vi "Begin.vi"(11 "Image Size":T1=enum."160x120") -> (0 "error out":errorcluster)   [LabVIEW 2012]
doc: "Called before other user functions, this VI is expected to open initial I/O refnums, load in file data, and do all program initialization. Notice that the <B>error out</B> terminal is simply used for data flow. Wiring it to other structures or subVIs ensures that this VI runs first."
uses:
  <vilib>/Rock Robotics/WPI/Camera/WPI_CameraImageSize.ctl
  <vilib>/Rock Robotics/WPI/Camera/WPI_CameraWhite Balance Values.ctl
  <vilib>/Rock Robotics/WPI/Camera/WPI_CameraExposure Values.ctl
  <vilib>/Rock Robotics/WPI/Camera/WPI_CameraFrameRate.ctl
  <vilib>/Rock Robotics/WPI/DriverStation/WPI_DriverStationRobotMode2.ctl
  <vilib>/Rock Robotics/SystemInterfaces/DIO/FPGA_DIOPWMChannel.ctl
  <vilib>/Rock Robotics/WPI/Joystick/WPI_JoystickDeviceEnum.ctl
  <vilib>/Rock Robotics/SystemInterfaces/Typedef/FPGA_TypedefDigitalModule.ctl
  <vilib>/Rock Robotics/WPI/Relay/WPI_RelayDirection.ctl
  <vilib>/Rock Robotics/SystemInterfaces/DIO/FPGA_DIORelayChannel.ctl
  <vilib>/Rock Robotics/SystemInterfaces/AI/FPGA_AIChannel.ctl
  <vilib>/Rock Robotics/SystemInterfaces/AI/FPGA_AIGyroChannel.ctl
  <vilib>/Rock Robotics/SystemInterfaces/DIO/FPGA_DIOChannel.ctl
  Robot Global Data.vi
  <vilib>/Rock Robotics/WPI/MotorControl/WPI_MotorControlOpen Victor.vi
  <vilib>/Rock Robotics/WPI/MotorControl/WPI_MotorControlOpen Jaguar.vi
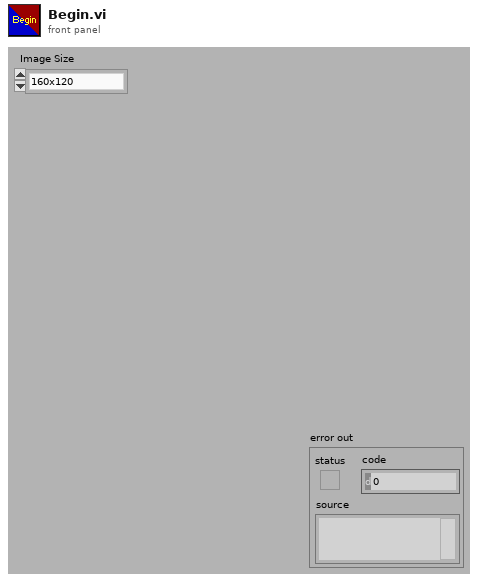
[diagram p1: front panel]
types:
  T1 = typedef "WPI_CameraImageSize.ctl" = enum16{"640x480", "320x240", "160x120"}
  T2 = typedef "FPGA_AIChannel.ctl" = enum8{"AI 1", "AI 2", "AI 3", "AI 4", "AI 5", "AI 6", "AI 7", "AI 8", "Invalid"}
  T3 = typedef "FPGA_DIOChannel.ctl" = enum8{"DIO 1", "DIO 2", "DIO 3", "DIO 4", "DIO 5", "DIO 6", "DIO 7", "DIO 8", "DIO 9", "DIO 10", "DIO 11", "DIO 12", "DIO 13", "DIO 14", "Invalid"}
  T4 = typedef "FPGA_TypedefDigitalModule.ctl" = enum16{"Digital Module 1", "Digital Module 2"}
  T5 = typedef "FPGA_DIOPWMChannel.ctl" = enum8{"PWM 1", "PWM 2", "PWM 3", "PWM 4", "PWM 5", "PWM 6", "PWM 7", "PWM 8", "PWM 9", "PWM 10", "Invalid"}
  T6 = typedef "FPGA_AIGyroChannel.ctl" = enum8{"AI 1", "AI 2", "Invalid"}
  T7 = typedef "FPGA_DIORelayChannel.ctl" = enum8{"Relay 1", "Relay 2", "Relay 3", "Relay 4", "Relay 5", "Relay 6", "Relay 7", "Relay 8", "Invalid"}
  T8 = typedef "WPI_RelayDirection.ctl" = enum16{"Both directions", "Forward only", "Reverse only"}
  T9 = typedef "WPI_JoystickDeviceEnum.ctl" = enum16{"USB 1", "USB 2", "USB 3", "USB 4", "Kinect 1", "Kinect 2"}
  T10 = typedef "WPI_DriverStationRobotMode2.ctl" = enum16{"Autonomous Disabled", "Autonomous Enabled", "Teleop Disabled", "Teleop Enabled", "Timeout", "Finish", "Test Disabled", "Test Enabled"}
  T11 = typedef "WPI_CameraFrameRate.ctl" = u32
  T12 = typedef "WPI_CameraExposure Values.ctl" = enum16{"Auto", "Flicker-free 50 Hz", "Flicker-free 60 Hz", "Hold current"}
  T13 = typedef "WPI_CameraWhite Balance Values.ctl" = enum16{"Auto", "Fixed indoor", "Fixed outdoor 1", "Fixed outdoor 2", "Fixed fluorescent 1", "Fixed fluorescent 2", "Hold current"}
  T14 = typedef "WPI_MotorControlDeviceRef.ctl" = cluster{"DeviceStatus":errorcluster, "Type":enum16{"PWM", "CAN"}, "PWM":cluster{"Digital Module":T4, "PWM Channel":T5, "DeadBand":T15}, "CAN":cluster{"Device Number":u8, "Control Mode":T16, "Semaphore":T17, "Max Vout":dbl}, "Invert":bool, "TransformRef":T18, "InvTransformRef":T18}
  T15 = typedef "WPI_PWMDeadband.ctl" = cluster{"Name":string, "maxPositivePwm":i32, "minPositivePwm":i32, "centerPwm":i32, "maxNegativePwm":i32, "minNegativePwm":i32, "angularRange":u16}
  T16 = typedef "WPI_CANJaguar_ControlMode.ctl" = enum8{"Percent VBus", "Current", "Speed", "Position", "Voltage"}
  T17 = typedef "Semaphore RefNum" = refnum<k1>
  T18 = typedef "WPI_PWMTransform_ConPane.ctl" = refnum<vi>
  T19 = typedef "WPI_CameraDevRef.ctl" = cluster{"Camera Address":string, "CameraStatus":errorcluster, "Acquire Image Notifier":refnum<notifier>}
  T20 = typedef "WPI_JoystickDevRef.ctl" = cluster{"Device":T9}
  T21 = typedef "WPI_ServoDeviceRef.ctl" = cluster{"DeviceStatus":errorcluster, "Digital Module":T4, "PWM Channel":T5, "DeadBand":T15}
  T22 = typedef "WPI_RelayDevRef.ctl" = cluster{"DevStatus":errorcluster, "Relay Channel":T7, "Digital Module":T4, "Relay Direction":T8}
  T23 = typedef "WPI_AnalogChannelDevRef.ctl" = cluster{"DevStatus":errorcluster, "Analog Module":T24, "Analog Channel":T2}
  T24 = typedef "FPGA_TypedefAnalogModule.ctl" = enum16{"Analog Module 1", "Analog Module 2"}
  T25 = typedef "WPI_DigitalInputDevRef.ctl" = cluster{"DevStatus":errorcluster, "DIO Channel":T3, "Digital Module":T4}
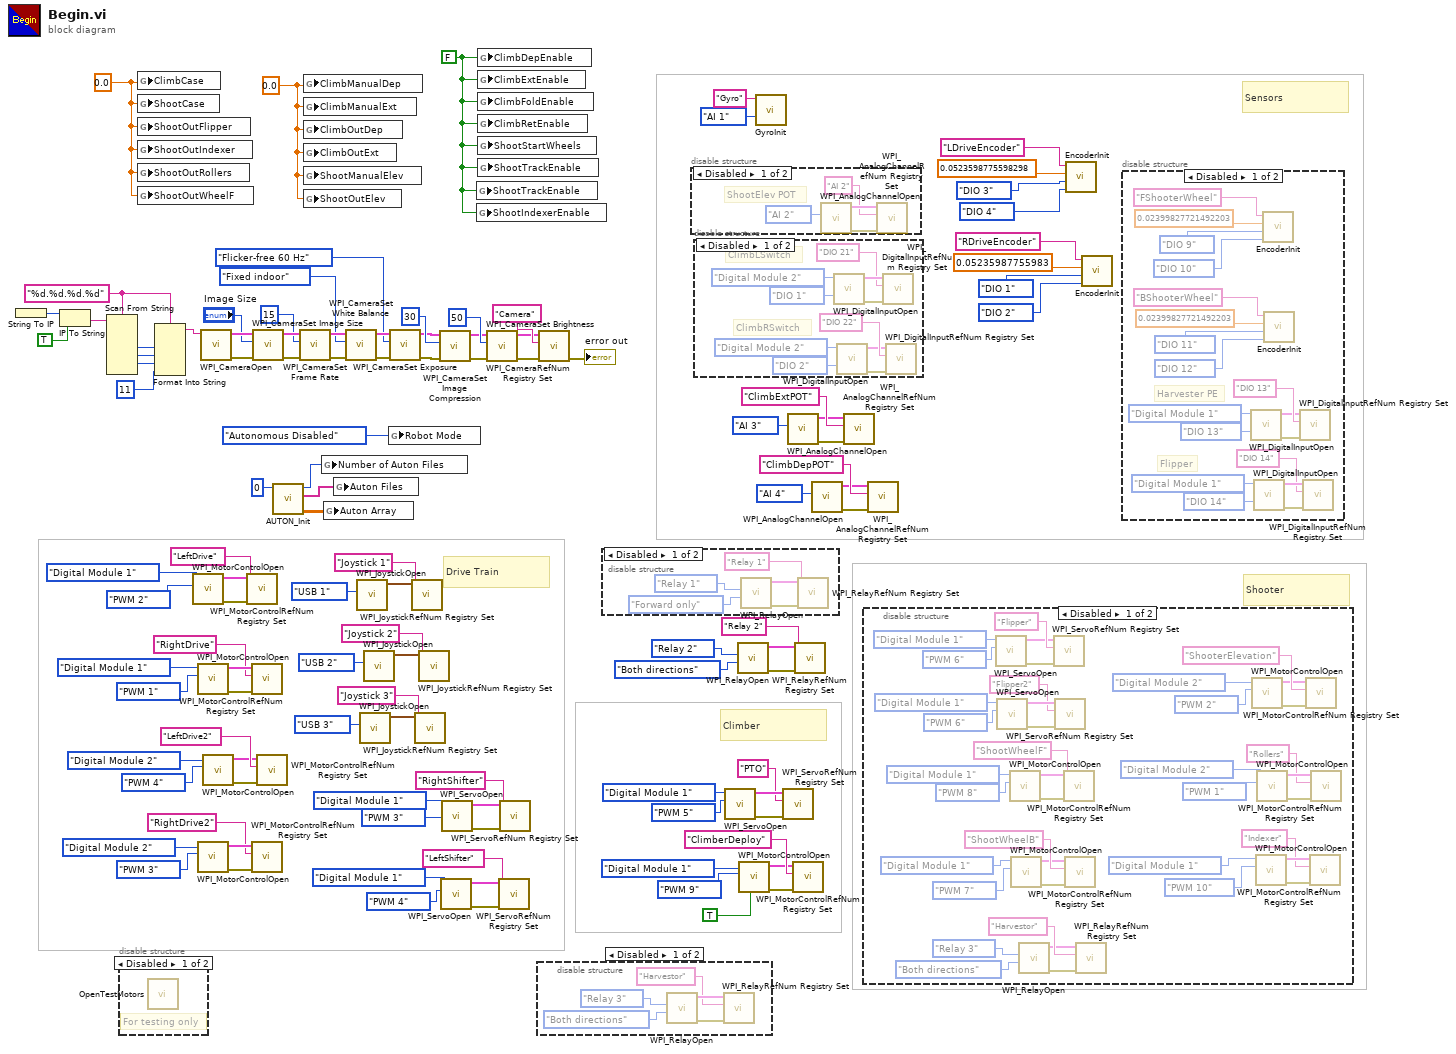
[diagram p0: block diagram]
diagram:
  w57 = FALSE ("ClimbDepEnable")
  w58 = 0.0 ("ClimbCase")
  w59 = 0.0 ("ClimbCase")
  w84 = "%d.%d.%d.%d" ("format string")
  # "Drive Train"
  # "Climber"
  # "Shooter"
  # "Sensors"
  n1 = String To IP() -> (0:w91:u32)  [unwired: 1 in]
  n2 = IP To String(1:TRUE ("dot notation? (F)"), 2:w91) -> (0:w89:string)
  n3 = Scan From String(format string=w84, input string=w89) -> (output 1=w88:i32, output 2=w87:i32, output 3=w86:i32)  [unwired: 7 in, 3 out]
  n4 = disable-structure shown="Disabled" {
    frame Disabled {
      # "For testing only"
      n5 = call "OpenTestMotors.vi"() -> ()  [unwired: 12 in]
    }
    frame Enabled {
    }
  }
  n6 = global write "Robot Global Data.vi" "ClimbCase"(w59) -> ()
  n7 = global write "Robot Global Data.vi" "ShootCase"(w59) -> ()
  n8 = global write "Robot Global Data.vi" "ShootOutFlipper"(w59) -> ()
  n9 = global write "Robot Global Data.vi" "ShootOutIndexer"(w59) -> ()
  n10 = global write "Robot Global Data.vi" "ShootOutRollers"(w59) -> ()
  n11 = global write "Robot Global Data.vi" "ShootOutWheelF"(w59) -> ()
  n12 = Format Into String(format string=w84, w88, w87, w86, 11 ("Compression")) -> (resulting string=w82:string)  [unwired: 2 in, 1 out]
  n13 = call-poly <vilib>:"WPI_MotorControlOpen.vi"("PWM Channel"=FPGA_DIOPWMChannel."PWM 2", "Digital Module (Module 1)"=FPGA_TypedefDigitalModule."Digital Module 1") -> ("error out"=w69:errorcluster, "MotorControlDeviceRef"=w70:T14)  [unwired: 8 in]
  n14 = call-poly <vilib>:"WPI_MotorControlOpen.vi"("PWM Channel"=FPGA_DIOPWMChannel."PWM 1", "Digital Module (Module 1)"=FPGA_TypedefDigitalModule."Digital Module 1") -> ("error out"=w76:errorcluster, "MotorControlDeviceRef"=w75:T14)  [unwired: 8 in]
  n15 = call-poly <vilib>:"WPI_MotorControlOpen.vi"("PWM Channel"=FPGA_DIOPWMChannel."PWM 3", "Digital Module (Module 1)"=FPGA_TypedefDigitalModule."Digital Module 2") -> ("error out"=w55:errorcluster, "MotorControlDeviceRef"=w54:T14)  [unwired: 8 in]
  n16 = call <vilib>:"WPI_CameraOpen.vi"("Camera Address"=w82) -> ("error out"=w103:errorcluster, "CameraDevRef"=w104:T19)  [unwired: 1 in, 8 out]
  n17 = call-poly <vilib>:"WPI_MotorControlOpen.vi"("PWM Channel"=FPGA_DIOPWMChannel."PWM 4", "Digital Module (Module 1)"=FPGA_TypedefDigitalModule."Digital Module 2") -> ("error out"=w46:errorcluster, "MotorControlDeviceRef"=w47:T14)  [unwired: 8 in]
  n18 = call <vilib>:"WPI_MotorControlRefNum Registry Set.vi"("error in (no error)"=w69, "refnum name"="LeftDrive", "MotorControlDevRef"=w70) -> ()  [unwired: 7 in, 2 out]
  n19 = call <vilib>:"WPI_MotorControlRefNum Registry Set.vi"("error in (no error)"=w76, "refnum name"="RightDrive", "MotorControlDevRef"=w75) -> ()  [unwired: 7 in, 2 out]
  n20 = call <vilib>:"WPI_MotorControlRefNum Registry Set.vi"("error in (no error)"=w55, "refnum name"="RightDrive2", "MotorControlDevRef"=w54) -> ()  [unwired: 7 in, 2 out]
  n21 = call <vilib>:"WPI_CameraSet Image Size.vi"("error in (no error)"=w103, "Image Size"="Image Size", "CameraDevRef"=w104) -> ("error out"=w102:errorcluster, "CameraDevRef Out"=w105:T19)  [unwired: 7 out]
  n22 = call <vilib>:"WPI_MotorControlRefNum Registry Set.vi"("error in (no error)"=w46, "refnum name"="LeftDrive2", "MotorControlDevRef"=w47) -> ()  [unwired: 7 in, 2 out]
  n23 = call "AUTON_Init.vi"("Default File"=0) -> ("Auton Array"=w77:dbl[][], "Auton Files"=w78:string[], "Number of Auton Files"=w79:i64)  [unwired: 8 in]
  n24 = call <vilib>:"WPI_CameraSet Frame Rate.vi"("error in (no error)"=w102, "Frame Rate (fps)"=T11 15, "CameraDevRef"=w105) -> ("error out"=w101:errorcluster, "CameraDevRef Out"=w107:T19)  [unwired: 7 out]
  n25 = global write "Robot Global Data.vi" "ClimbManualDep"(w58) -> ()
  n26 = global write "Robot Global Data.vi" "ClimbManualExt"(w58) -> ()
  n27 = global write "Robot Global Data.vi" "ClimbOutDep"(w58) -> ()
  n28 = global write "Robot Global Data.vi" "ClimbOutExt"(w58) -> ()
  n29 = global write "Robot Global Data.vi" "ShootManualElev"(w58) -> ()
  n30 = global write "Robot Global Data.vi" "ShootOutElev"(w58) -> ()
  n31 = global write "Robot Global Data.vi" "Number of Auton Files"(w79) -> ()
  n32 = global write "Robot Global Data.vi" "Auton Array"(w77) -> ()
  n33 = global write "Robot Global Data.vi" "Auton Files"(w78) -> ()
  n34 = call <vilib>:"WPI_CameraSet White Balance.vi"("error in (no error)"=w101, "White Balance"=WPI_CameraWhite_Balance_Values."Fixed indoor", "CameraDevRef"=w107) -> ("error out"=w100:errorcluster, "CameraDevRef Out"=w106:T19)  [unwired: 7 out]
  n35 = call <vilib>:"WPI_JoystickOpen.vi"("JoystickDevice"=WPI_JoystickDeviceEnum."USB 1") -> ("JoystickDevRef"=w60:T20)  [unwired: 10 in]
  n36 = call <vilib>:"WPI_JoystickOpen.vi"("JoystickDevice"=WPI_JoystickDeviceEnum."USB 3") -> ("JoystickDevRef"=w66:T20)  [unwired: 10 in]
  n37 = call <vilib>:"WPI_JoystickOpen.vi"("JoystickDevice"=WPI_JoystickDeviceEnum."USB 2") -> ("JoystickDevRef"=w65:T20)  [unwired: 10 in]
  n38 = global write "Robot Global Data.vi" "Robot Mode"(WPI_DriverStationRobotMode2."Autonomous Disabled" ("Robot Mode")) -> ()
  n39 = call <vilib>:"WPI_CameraSet Exposure.vi"("error in (no error)"=w100, "Exposure"=WPI_CameraExposure_Values."Flicker-free 60 Hz", "CameraDevRef"=w106) -> ("error out"=w99:errorcluster, "CameraDevRef Out"=w109:T19)  [unwired: 7 out]
  n40 = call <vilib>:"WPI_JoystickRefNum Registry Set.vi"("refnum name"="Joystick 1", "JoystickDevRef"=w60) -> ()  [unwired: 8 in, 2 out]
  n41 = call <vilib>:"WPI_JoystickRefNum Registry Set.vi"("refnum name"="Joystick 3", "JoystickDevRef"=w66) -> ()  [unwired: 8 in, 2 out]
  n42 = call <vilib>:"WPI_JoystickRefNum Registry Set.vi"("refnum name"="Joystick 2", "JoystickDevRef"=w65) -> ()  [unwired: 8 in, 2 out]
  n43 = call <vilib>:"WPI_CameraSet Image Compression.vi"("error in (no error)"=w99, "Compression"=30, "CameraDevRef"=w109) -> ("error out"=w98:errorcluster, "CameraDevRef Out"=w108:T19)  [unwired: 7 out]
  n44 = call <vilib>:"WPI_ServoOpen.vi"("PWM Channel"=FPGA_DIOPWMChannel."PWM 4", "Digital Module (Module 1)"=FPGA_TypedefDigitalModule."Digital Module 1") -> ("error out"=w39:errorcluster, "ServoDeviceRef"=w32:T21)  [unwired: 8 in]
  n45 = call <vilib>:"WPI_ServoOpen.vi"("PWM Channel"=FPGA_DIOPWMChannel."PWM 3", "Digital Module (Module 1)"=FPGA_TypedefDigitalModule."Digital Module 1") -> ("error out"=w38:errorcluster, "ServoDeviceRef"=w37:T21)  [unwired: 8 in]
  n46 = global write "Robot Global Data.vi" "ShootTrackEnable"(w57) -> ()
  n47 = global write "Robot Global Data.vi" "ShootIndexerEnable"(w57) -> ()
  n48 = global write "Robot Global Data.vi" "ClimbDepEnable"(w57) -> ()
  n49 = global write "Robot Global Data.vi" "ClimbExtEnable"(w57) -> ()
  n50 = global write "Robot Global Data.vi" "ClimbFoldEnable"(w57) -> ()
  n51 = global write "Robot Global Data.vi" "ClimbRetEnable"(w57) -> ()
  n52 = global write "Robot Global Data.vi" "ShootStartWheels"(w57) -> ()
  n53 = global write "Robot Global Data.vi" "ShootTrackEnable"(w57) -> ()
  n54 = call <vilib>:"WPI_CameraSet Brightness.vi"("error in (no error)"=w98, "Brightness"=50, "CameraDevRef"=w108) -> ("error out"=w96:errorcluster, "CameraDevRef Out"=w97:T19)  [unwired: 7 out]
  n55 = call <vilib>:"WPI_ServoRefNum Registry Set.vi"("error in (no error)"=w39, "refnum name"="LeftShifter", "ServoDeviceRef"=w32) -> ()  [unwired: 7 in, 2 out]
  n56 = call <vilib>:"WPI_ServoRefNum Registry Set.vi"("error in (no error)"=w38, "refnum name"="RightShifter", "ServoDeviceRef"=w37) -> ()  [unwired: 7 in, 2 out]
  n57 = disable-structure shown="Disabled" {
    frame Disabled {
      n58 = call <vilib>:"WPI_RelayOpen.vi"("Relay Direction"=WPI_RelayDirection."Both directions", "Relay Channel"=FPGA_DIORelayChannel."Relay 3") -> ("error out"=w117:errorcluster, "RelayDevRef"=w116:T22)  [unwired: 8 in]
      n59 = call <vilib>:"WPI_RelayRefNum Registry Set.vi"("error in (no error)"=w117, "refnum name"="Harvestor", "RelayDevRef"=w116) -> ()  [unwired: 7 in, 2 out]
    }
    frame Enabled {
    }
  }
  n60 = call <vilib>:"WPI_CameraRefNum Registry Set.vi"("error in (no error)"=w96, "refnum name"="Camera", "CameraDevRef"=w97) -> ("error out"=→"error out":errorcluster)  [unwired: 8 out]
  n61 = disable-structure shown="Disabled" {
    frame Disabled {
      n62 = call <vilib>:"WPI_RelayOpen.vi"("Relay Direction"=WPI_RelayDirection."Forward only", "Relay Channel"=FPGA_DIORelayChannel."Relay 1") -> ("error out"=w122:errorcluster, "RelayDevRef"=w121:T22)  [unwired: 8 in]
      n63 = call <vilib>:"WPI_RelayRefNum Registry Set.vi"("error in (no error)"=w122, "refnum name"="Relay 1", "RelayDevRef"=w121) -> ()  [unwired: 7 in, 2 out]
    }
    frame Enabled {
    }
  }
  n64 = disable-structure shown="Disabled" {
    frame Disabled {
      # "ShootElev POT"
      n65 = call <vilib>:"WPI_AnalogChannelOpen.vi"("Analog Channel"=FPGA_AIChannel."AI 2") -> ("error out"=w123:errorcluster, "AIDeviceRef"=w125:T23)  [unwired: 9 in]
      n66 = call <vilib>:"WPI_AnalogChannelRefNum Registry Set.vi"("error in (no error)"=w123, "refnum name"="AI 2", "AIDeviceRef"=w125) -> ()  [unwired: 7 in, 2 out]
    }
    frame Enabled {
    }
  }
  n67 = disable-structure shown="Disabled" {
    frame Disabled {
      # "ClimbRSwitch"
      # "ClimbLSwitch"
      n68 = call <vilib>:"WPI_DigitalInputOpen.vi"("DIO Channel"=FPGA_DIOChannel."DIO 1", "Digital Module (Module 1)"=FPGA_TypedefDigitalModule."Digital Module 2") -> ("error out"=w128:errorcluster, "DigitalInputDevRef"=w129:T25)  [unwired: 8 in]
      n69 = call <vilib>:"WPI_DigitalInputOpen.vi"("DIO Channel"=FPGA_DIOChannel."DIO 2", "Digital Module (Module 1)"=FPGA_TypedefDigitalModule."Digital Module 2") -> ("error out"=w135:errorcluster, "DigitalInputDevRef"=w134:T25)  [unwired: 8 in]
      n70 = call <vilib>:"WPI_DigitalInputRefNum Registry Set.vi"("error in (no error)"=w128, "refnum name"="DIO 21", "DigitalInputDevRef"=w129) -> ()  [unwired: 7 in, 2 out]
      n71 = call <vilib>:"WPI_DigitalInputRefNum Registry Set.vi"("error in (no error)"=w135, "refnum name"="DIO 22", "DigitalInputDevRef"=w134) -> ()  [unwired: 7 in, 2 out]
    }
    frame Enabled {
    }
  }
  n72 = call <vilib>:"WPI_ServoOpen.vi"("PWM Channel"=FPGA_DIOPWMChannel."PWM 5", "Digital Module (Module 1)"=FPGA_TypedefDigitalModule."Digital Module 1") -> ("error out"=w17:errorcluster, "ServoDeviceRef"=w16:T21)  [unwired: 8 in]
  n73 = call <vilib>:"WPI_RelayOpen.vi"("Relay Direction"=WPI_RelayDirection."Both directions", "Relay Channel"=FPGA_DIORelayChannel."Relay 2") -> ("error out"=w40:errorcluster, "RelayDevRef"=w41:T22)  [unwired: 8 in]
  n74 = call-poly <vilib>:"WPI_MotorControlOpen.vi"("Invert"=TRUE, "PWM Channel"=FPGA_DIOPWMChannel."PWM 9", "Digital Module (Module 1)"=FPGA_TypedefDigitalModule."Digital Module 1") -> ("error out"=w22:errorcluster, "MotorControlDeviceRef"=w21:T14)  [unwired: 7 in]
  n75 = call "GyroInit.vi"("refnum name"="Gyro", "Analog Channel"=FPGA_AIGyroChannel."AI 1") -> ()  [unwired: 8 in]
  n76 = call <vilib>:"WPI_ServoRefNum Registry Set.vi"("error in (no error)"=w17, "refnum name"="PTO", "ServoDeviceRef"=w16) -> ()  [unwired: 7 in, 2 out]
  n77 = call <vilib>:"WPI_AnalogChannelOpen.vi"("Analog Channel"=FPGA_AIChannel."AI 3") -> ("error out"=w1:errorcluster, "AIDeviceRef"=w2:T23)  [unwired: 9 in]
  n78 = call <vilib>:"WPI_MotorControlRefNum Registry Set.vi"("error in (no error)"=w22, "refnum name"="ClimberDeploy", "MotorControlDevRef"=w21) -> ()  [unwired: 7 in, 2 out]
  n79 = call <vilib>:"WPI_RelayRefNum Registry Set.vi"("error in (no error)"=w40, "refnum name"="Relay 2", "RelayDevRef"=w41) -> ()  [unwired: 7 in, 2 out]
  n80 = call <vilib>:"WPI_AnalogChannelOpen.vi"("Analog Channel"=FPGA_AIChannel."AI 4") -> ("error out"=w26:errorcluster, "AIDeviceRef"=w27:T23)  [unwired: 9 in]
  n81 = call <vilib>:"WPI_AnalogChannelRefNum Registry Set.vi"("error in (no error)"=w1, "refnum name"="ClimbExtPOT", "AIDeviceRef"=w2) -> ()  [unwired: 7 in, 2 out]
  n82 = disable-structure shown="Disabled" {
    frame Disabled {
      n83 = call <vilib>:"WPI_ServoOpen.vi"("PWM Channel"=FPGA_DIOPWMChannel."PWM 6", "Digital Module (Module 1)"=FPGA_TypedefDigitalModule."Digital Module 1") -> ("error out"=w152:errorcluster, "ServoDeviceRef"=w153:T21)  [unwired: 8 in]
      n84 = call <vilib>:"WPI_ServoOpen.vi"("PWM Channel"=FPGA_DIOPWMChannel."PWM 6", "Digital Module (Module 1)"=FPGA_TypedefDigitalModule."Digital Module 1") -> ("error out"=w146:errorcluster, "ServoDeviceRef"=w145:T21)  [unwired: 8 in]
      n85 = call-poly <vilib>:"WPI_MotorControlOpen.vi"("PWM Channel"=FPGA_DIOPWMChannel."PWM 8", "Digital Module (Module 1)"=FPGA_TypedefDigitalModule."Digital Module 1") -> ("error out"=w163:errorcluster, "MotorControlDeviceRef"=w164:T14)  [unwired: 8 in]
      n86 = call-poly <vilib>:"WPI_MotorControlOpen.vi"("PWM Channel"=FPGA_DIOPWMChannel."PWM 7", "Digital Module (Module 1)"=FPGA_TypedefDigitalModule."Digital Module 1") -> ("error out"=w149:errorcluster, "MotorControlDeviceRef"=w148:T14)  [unwired: 8 in]
      n87 = call <vilib>:"WPI_RelayOpen.vi"("Relay Direction"=WPI_RelayDirection."Both directions", "Relay Channel"=FPGA_DIORelayChannel."Relay 3") -> ("error out"=w137:errorcluster, "RelayDevRef"=w138:T22)  [unwired: 8 in]
      n88 = call <vilib>:"WPI_ServoRefNum Registry Set.vi"("error in (no error)"=w152, "refnum name"="Flipper", "ServoDeviceRef"=w153) -> ()  [unwired: 7 in, 2 out]
      n89 = call <vilib>:"WPI_ServoRefNum Registry Set.vi"("error in (no error)"=w146, "refnum name"="Flipper2", "ServoDeviceRef"=w145) -> ()  [unwired: 7 in, 2 out]
      n90 = call <vilib>:"WPI_MotorControlRefNum Registry Set.vi"("error in (no error)"=w163, "refnum name"="ShootWheelF", "MotorControlDevRef"=w164) -> ()  [unwired: 7 in, 2 out]
      n91 = call <vilib>:"WPI_MotorControlRefNum Registry Set.vi"("error in (no error)"=w149, "refnum name"="ShootWheelB", "MotorControlDevRef"=w148) -> ()  [unwired: 7 in, 2 out]
      n92 = call <vilib>:"WPI_RelayRefNum Registry Set.vi"("error in (no error)"=w137, "refnum name"="Harvestor", "RelayDevRef"=w138) -> ()  [unwired: 7 in, 2 out]
      n93 = call-poly <vilib>:"WPI_MotorControlOpen.vi"("PWM Channel"=FPGA_DIOPWMChannel."PWM 2", "Digital Module (Module 1)"=FPGA_TypedefDigitalModule."Digital Module 2") -> ("error out"=w174:errorcluster, "MotorControlDeviceRef"=w173:T14)  [unwired: 8 in]
      n94 = call-poly <vilib>:"WPI_MotorControlOpen.vi"("PWM Channel"=FPGA_DIOPWMChannel."PWM 10", "Digital Module (Module 1)"=FPGA_TypedefDigitalModule."Digital Module 1") -> ("error out"=w159:errorcluster, "MotorControlDeviceRef"=w160:T14)  [unwired: 8 in]
      n95 = call-poly <vilib>:"WPI_MotorControlOpen.vi"("PWM Channel"=FPGA_DIOPWMChannel."PWM 1", "Digital Module (Module 1)"=FPGA_TypedefDigitalModule."Digital Module 2") -> ("error out"=w169:errorcluster, "MotorControlDeviceRef"=w170:T14)  [unwired: 8 in]
      n96 = call <vilib>:"WPI_MotorControlRefNum Registry Set.vi"("error in (no error)"=w174, "refnum name"="ShooterElevation", "MotorControlDevRef"=w173) -> ()  [unwired: 7 in, 2 out]
      n97 = call <vilib>:"WPI_MotorControlRefNum Registry Set.vi"("error in (no error)"=w159, "refnum name"="Indexer", "MotorControlDevRef"=w160) -> ()  [unwired: 7 in, 2 out]
      n98 = call <vilib>:"WPI_MotorControlRefNum Registry Set.vi"("error in (no error)"=w169, "refnum name"="Rollers", "MotorControlDevRef"=w170) -> ()  [unwired: 7 in, 2 out]
    }
    frame Enabled {
    }
  }
  n99 = call <vilib>:"WPI_AnalogChannelRefNum Registry Set.vi"("error in (no error)"=w26, "refnum name"="ClimbDepPOT", "AIDeviceRef"=w27) -> ()  [unwired: 7 in, 2 out]
  n100 = call "EncoderInit.vi"("refnum name"="LDriveEncoder", "DistancePerCount"=0.0523598775598298, "DIO Channel"=FPGA_DIOChannel."DIO 3", "DIO Channel 2"=FPGA_DIOChannel."DIO 4") -> ()  [unwired: 7 in]
  n101 = call "EncoderInit.vi"("refnum name"="RDriveEncoder", "DistancePerCount"=0.05235987755983, "DIO Channel"=FPGA_DIOChannel."DIO 1", "DIO Channel 2"=FPGA_DIOChannel."DIO 2") -> ()  [unwired: 7 in]
  n102 = disable-structure shown="Disabled" {
    frame Disabled {
      # "Flipper"
      # "Harvester PE"
      n103 = call <vilib>:"WPI_DigitalInputOpen.vi"("DIO Channel"=FPGA_DIOChannel."DIO 13", "Digital Module (Module 1)"=FPGA_TypedefDigitalModule."Digital Module 1") -> ("error out"=w185:errorcluster, "DigitalInputDevRef"=w184:T25)  [unwired: 8 in]
      n104 = call <vilib>:"WPI_DigitalInputOpen.vi"("DIO Channel"=FPGA_DIOChannel."DIO 14", "Digital Module (Module 1)"=FPGA_TypedefDigitalModule."Digital Module 1") -> ("error out"=w178:errorcluster, "DigitalInputDevRef"=w179:T25)  [unwired: 8 in]
      n105 = call "EncoderInit.vi"("refnum name"="FShooterWheel", "DistancePerCount"=0.02399827721492203, "DIO Channel"=FPGA_DIOChannel."DIO 9", "DIO Channel 2"=FPGA_DIOChannel."DIO 10") -> ()  [unwired: 7 in]
      n106 = call "EncoderInit.vi"("refnum name"="BShooterWheel", "DistancePerCount"=0.02399827721492203, "DIO Channel"=FPGA_DIOChannel."DIO 11", "DIO Channel 2"=FPGA_DIOChannel."DIO 12") -> ()  [unwired: 7 in]
      n107 = call <vilib>:"WPI_DigitalInputRefNum Registry Set.vi"("error in (no error)"=w185, "refnum name"="DIO 13", "DigitalInputDevRef"=w184) -> ()  [unwired: 7 in, 2 out]
      n108 = call <vilib>:"WPI_DigitalInputRefNum Registry Set.vi"("error in (no error)"=w178, "refnum name"="DIO 14", "DigitalInputDevRef"=w179) -> ()  [unwired: 7 in, 2 out]
    }
    frame Enabled {
    }
  }
